vi "PS4 Controller - Polling Read.vi"() -> ()   [LabVIEW 2011, in "LVH-PS4.lvlib"]
doc: "This example demonstrates how to read from a Play Station 4 controller using polling."
uses:
  vi.lib/LabVIEW Hacker/PS4-Controller/LVH-PS4.lvlib
  vi.lib/LabVIEW Hacker/PS4-Controller/Private/Type Defs/Indicators/Controller.ctl
  vi.lib/LabVIEW Hacker/PS4-Controller/Private/Type Defs/Indicators/Square.ctl
  vi.lib/LabVIEW Hacker/PS4-Controller/Private/Type Defs/Indicators/X.ctl
  vi.lib/LabVIEW Hacker/PS4-Controller/Private/Type Defs/Indicators/Circle.ctl
  vi.lib/LabVIEW Hacker/PS4-Controller/Private/Type Defs/Indicators/Triangle.ctl
  vi.lib/LabVIEW Hacker/PS4-Controller/Private/Type Defs/Indicators/L1.ctl
  vi.lib/LabVIEW Hacker/PS4-Controller/Private/Type Defs/Indicators/R1.ctl
  vi.lib/LabVIEW Hacker/PS4-Controller/Private/Type Defs/Indicators/Share.ctl
  vi.lib/LabVIEW Hacker/PS4-Controller/Private/Type Defs/Indicators/Options.ctl
  vi.lib/LabVIEW Hacker/PS4-Controller/Private/Type Defs/Indicators/PS.ctl
  vi.lib/LabVIEW Hacker/PS4-Controller/Private/Type Defs/Indicators/Pad_Button.ctl
  vi.lib/LabVIEW Hacker/PS4-Controller/Private/Type Defs/Indicators/Dpad.ctl
  vi.lib/LabVIEW Hacker/PS4-Controller/Private/Type Defs/Indicators/Slider.ctl
panel:
  out "PS4 Controller":T1={"Square Button"=FALSE, "X Button"=FALSE, "Circle Button"=FALSE, "Triangle Button"=FALSE, "L1"=FALSE, "R1"=FALSE, "Share Button"=FALSE, "Options Button"=FALSE, "PS Button"=FALSE, "Pad Button"=FALSE, "D-Pad"=5, "L2"=0, "R2"=0, "Thumbstick_Left"={[], []}, "Thumbstick_Right"={[], []}} {"R2" scale=-32768.0..32767.0; "L2" scale=-32768.0..32767.0}
  in  "PS4 Controller Index":i32
  in  "Stop Button":bool
  # "Configure"
  # "Controller Data"
  # "PS4 Controller  - Polling Read\n\nThis example demonstrates how to read all button and axis data from a PS4 controller using a polling method.\n\nInstructions\n1. Select the Device Index associated with the PS4 Controller.     \n2. Click the Run Arrow.\n3. Notice the controller icon on the front panel update to match the actual controller state."
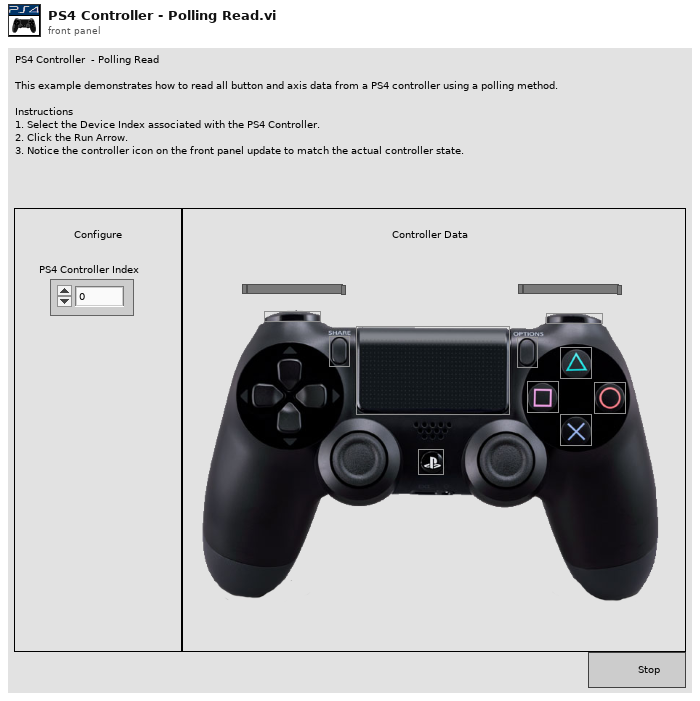
[diagram p1: front panel]
types:
  T1 = typedef "LVH-PS4.lvlib/Controller.ctl" = cluster{"Square Button":T2, "X Button":T3, "Circle Button":T4, "Triangle Button":T5, "L1":T6, "R1":T7, "Share Button":T8, "Options Button":T9, "PS Button":T10, "Pad Button":T11, "D-Pad":T12, "L2":T13, "R2":T13, "Thumbstick_Left":cluster{i32[], i32[]}, "Thumbstick_Right":cluster{i32[], i32[]}}
  T2 = typedef "LVH-PS4.lvlib/Square.ctl" = bool
  T3 = typedef "LVH-PS4.lvlib/X.ctl" = bool
  T4 = typedef "LVH-PS4.lvlib/Circle.ctl" = bool
  T5 = typedef "LVH-PS4.lvlib/Triangle.ctl" = bool
  T6 = typedef "LVH-PS4.lvlib/L1.ctl" = bool
  T7 = typedef "LVH-PS4.lvlib/R1.ctl" = bool
  T8 = typedef "LVH-PS4.lvlib/Share.ctl" = bool
  T9 = typedef "LVH-PS4.lvlib/Options.ctl" = bool
  T10 = typedef "LVH-PS4.lvlib/PS.ctl" = bool
  T11 = typedef "LVH-PS4.lvlib/Pad_Button.ctl" = bool
  T12 = typedef "LVH-PS4.lvlib/Dpad.ctl" = u16
  T13 = typedef "LVH-PS4.lvlib/Slider.ctl" = i32
  T14 = typedef "LVH-PS4.lvlib/PS4 Controller Ref.ctl" = cluster{"Controller Ref":refnum<k1>, "PS4 Events Ref":refnum<event-registration>, "Worker Ref":refnum<vi>}
  T15 = typedef "LVH-PS4.lvlib/Axis.ctl" = cluster{"Left Thumbstick":cluster{"X Axis":i32, "Y Axis":i32}, "Right Thumbstick":cluster{"X Axis":i32, "Y Axis":i32}, "L2":i32, "R2":i32, "D-Pad":T16}
  T16 = typedef "LVH-PS4.lvlib/DPad Enum.ctl" = enum16{"Idle", "Up", "Up / Right", "Right", "Down / Right", "Down", "Down / Left", "Left", "Up / Left"}
  T17 = typedef "LVH-PS4.lvlib/Buttons.ctl" = cluster{"Square":bool, "X":bool, "Circle":bool, "Triangle":bool, "L1":bool, "R1":bool, "L2":bool, "R2":bool, "Share":bool, "Options":bool, "Left Thumbstick":bool, "Right Thumbstick":bool, "Playstation Button":bool, "Pad":bool}
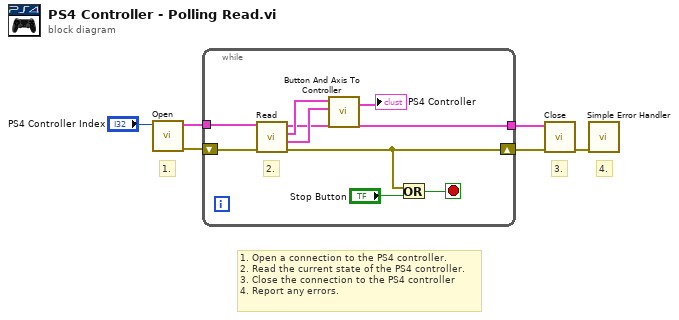
[diagram p0: block diagram]
diagram:
  # "1. Open a connection to the PS4 controller.\n2. Read the current state of the PS4 controller.\n3. Close the connection to the PS4 controller\n4. Report any errors."
  # "4."
  # "3."
  # "1."
  n1 = call "Open.vi"("Device Index"="PS4 Controller Index") -> ("Error Out"=w3:errorcluster, "PS4 Controller Ref"=w2:T14)  [unwired: 8 in, 1 out]
  n2 = while {
    shift-right: [w11] -> w6
    shift-left: w3 -> [w8]
    tunnel: [w10] -> w4
    tunnel: w2 -> [w9]
    stop <- w13 stop-if-true
    # "2."
    n3 = call "Read.vi"("Error In"=w8, "PS4 Controller Ref"=w9) -> ("Error Out"=w11:errorcluster, "All Axis"=w15:T15, "Buttons"=w14:T17, "PS4 Controller Ref"=w10:T14)  [unwired: 6 in]
    n4 = call "Button And Axis To Controller.vi"("All Axis"=w15, "Buttons"=w14) -> ("PS4 Controller"=→"PS4 Controller":T1)  [unwired: 5 in]
    n5 = Or(x=w11, y="Stop Button") -> (x .or. y?=w13:bool)
  }
  n6 = call "Close.vi"("Error In"=w6, "PS4 Controller Ref"=w4) -> ("Error Out"=w5:errorcluster)  [unwired: 9 in]
  n7 = call <vilib>:"Simple Error Handler.vi"("error in (no error)"=w5) -> ()  [unwired: 4 in, 5 out]
